vi "EQE_Park.vi"() -> (0 "Park":i32)   [LabVIEW 2017]
uses:
  Program Files (x86)/Bentham/SDK/code examples/LabView/8.0/BenHw/benhw32_stdcall.dll
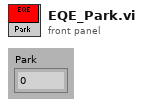
[diagram p1: front panel]
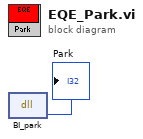
[diagram p0: block diagram]
diagram:
  n1 = dll-call lib="C:/Program Files (x86)/Bentham/SDK/code examples/LabView/8.0/BenHw/benhw32_stdcall.dll" fn="BI_park"() -> ("return type"=→"Park":i16)  [unwired: 3 in, 2 out]
